vi "create_data_file.vi"   [LabVIEW 2019]
uses:
  Global Variables/global.vi
  Instrument_Setup.vi
  Global Variables/Data_Display_global.vi
  Global Variables/Heat_global_variables.vi
types:
  T1 = enum16{"open", "replace", "create", "open or create", "replace or create", "replace or create with confirmation"}
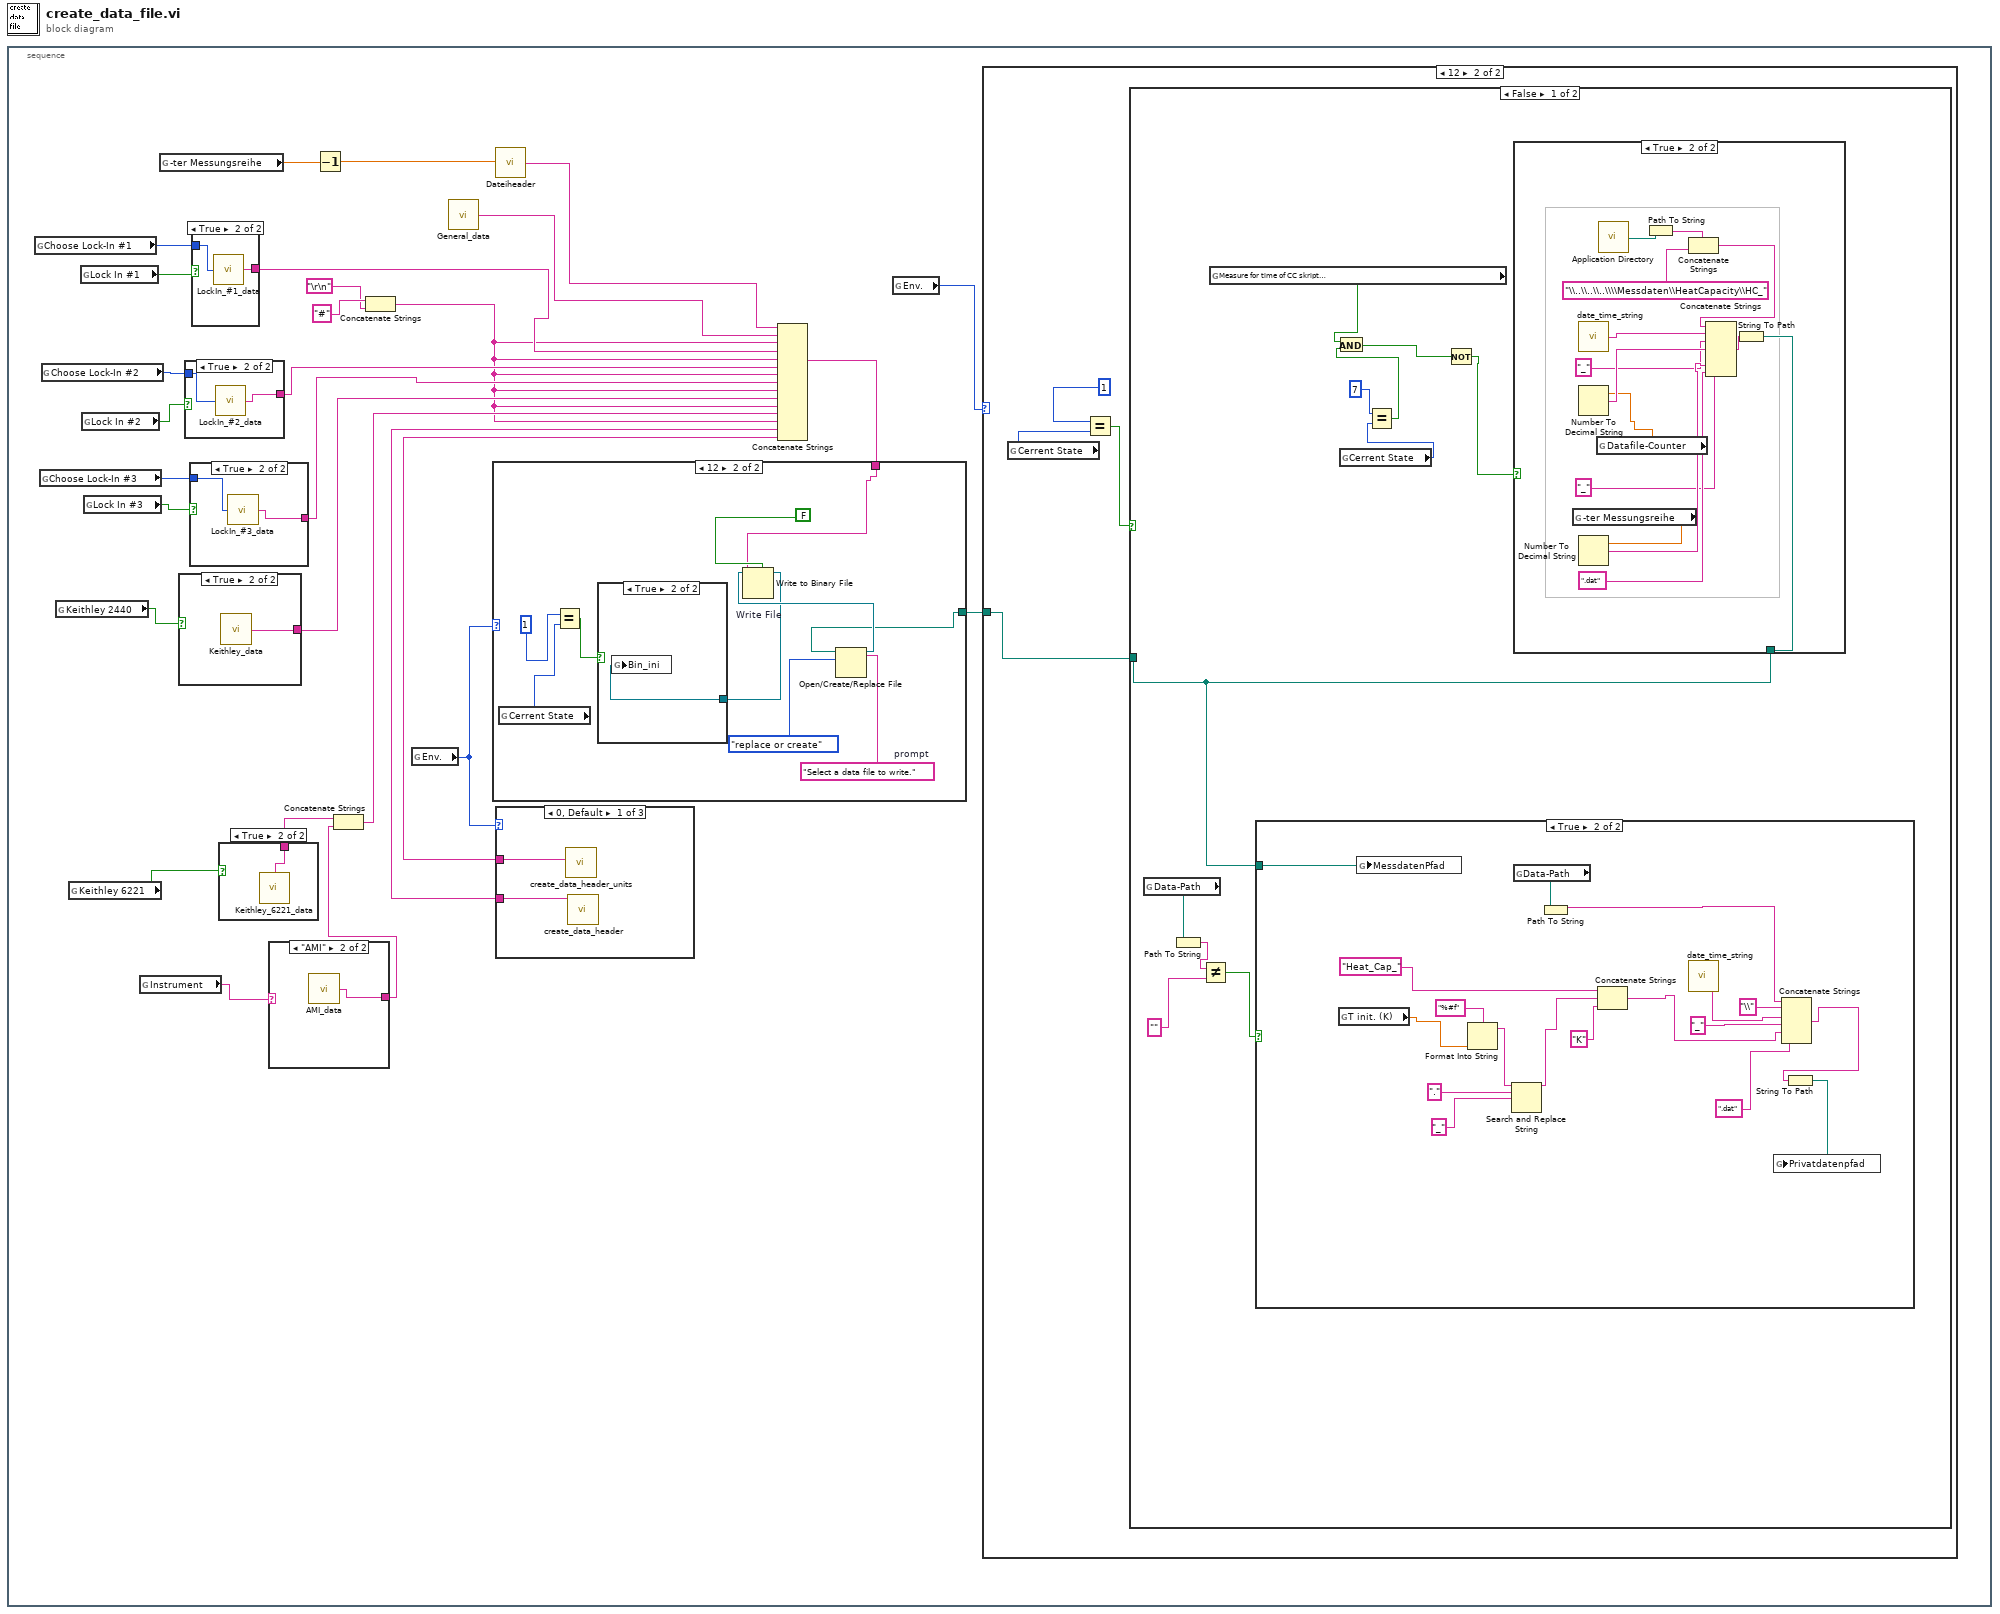
[diagram p0: block diagram]
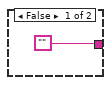
[diagram p2: hidden frame]
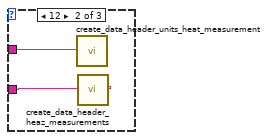
[diagram p3: hidden frame]
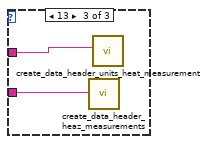
[diagram p4: hidden frame]
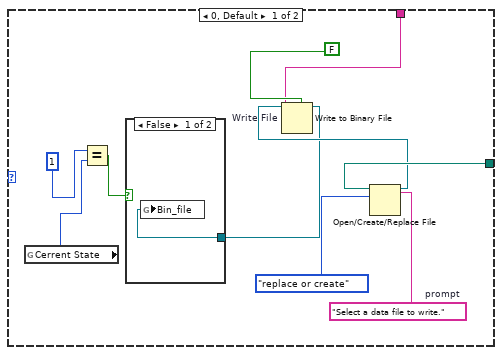
[diagram p5: hidden frame]
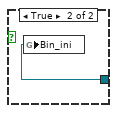
[diagram p6: hidden frame]
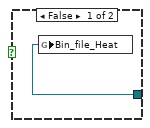
[diagram p7: hidden frame]
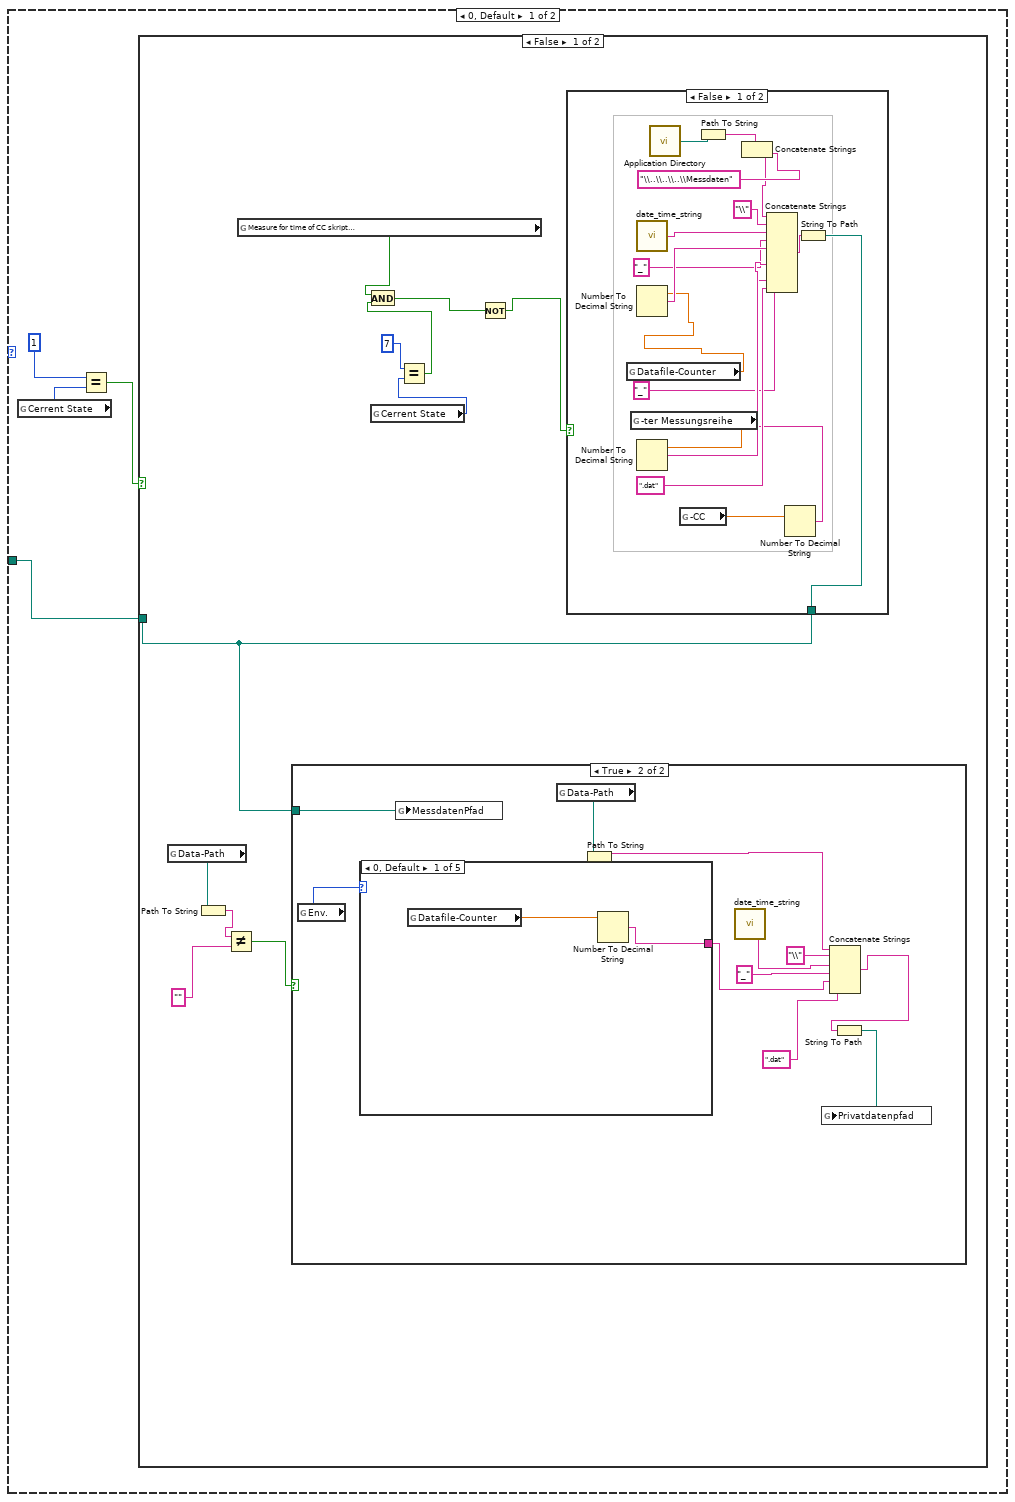
[diagram p8: hidden frame]
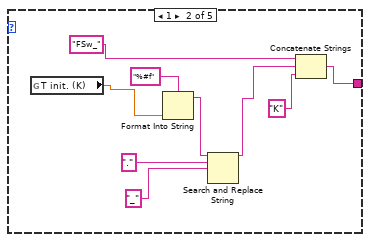
[diagram p10: hidden frame]
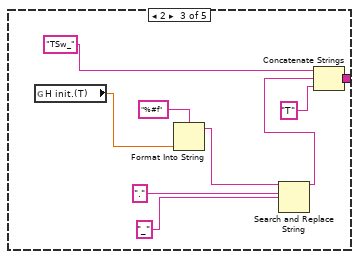
[diagram p11: hidden frame]
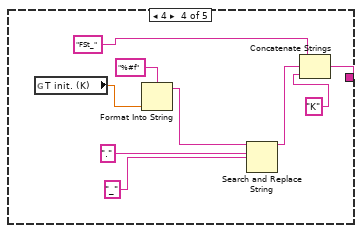
[diagram p12: hidden frame]
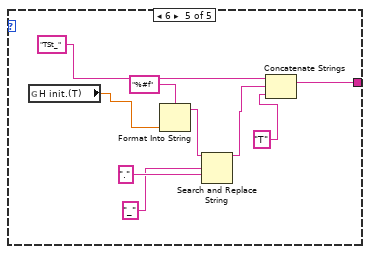
[diagram p13: hidden frame]
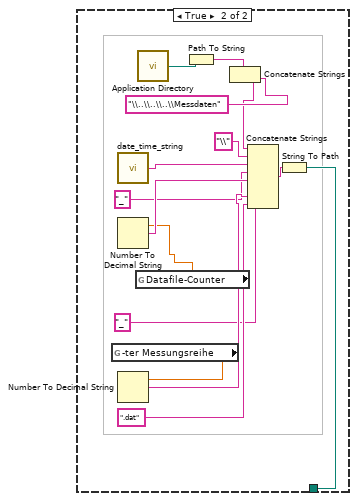
[diagram p14: hidden frame]
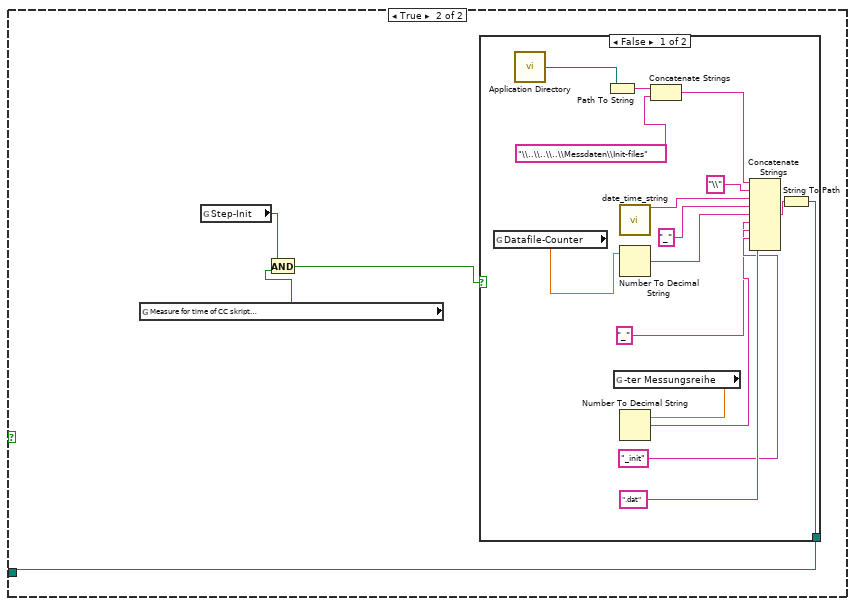
[diagram p15: hidden frame]
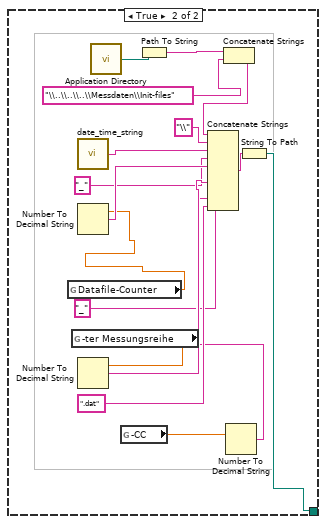
[diagram p16: hidden frame]
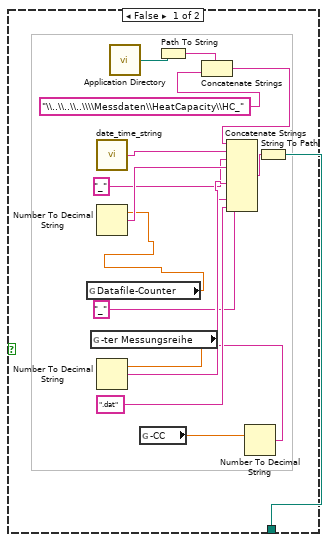
[diagram p18: hidden frame]
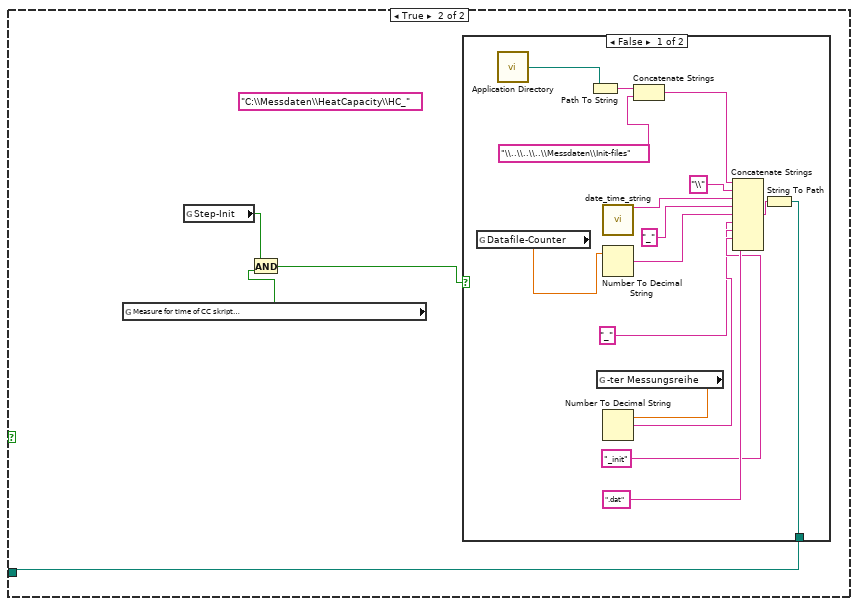
[diagram p19: hidden frame]
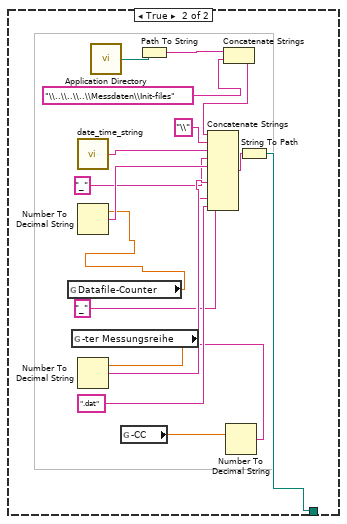
[diagram p20: hidden frame]
diagram:
  n1 = stacked-sequence {
    frame #0 {
      n2 = global read "Instrument_Setup.vi" "Choose Lock-In #1"() -> (w10:u16)
      n3 = global read "Instrument_Setup.vi" "Choose Lock-In #3"() -> (w7:u16)
      n4 = global read "Instrument_Setup.vi" "Choose Lock-In #2"() -> (w8:u16)
      n5 = global read "Instrument_Setup.vi" "Keithley 2440"() -> (w4:bool)
      n6 = global read "Instrument_Setup.vi" "Keithley 6221"() -> (w18:bool)
      n7 = global read "Instrument_Setup.vi" "Lock In #1"() -> (w21:bool)
      n8 = global read "Instrument_Setup.vi" "Lock In #2"() -> (w20:bool)
      n9 = global read "Instrument_Setup.vi" "Lock In #3"() -> (w12:bool)
      n10 = global read "Instrument_Setup.vi" "Instrument"() -> (w17:string)
      n11 = global read "global.vi" "-ter Messungsreihe"() -> (w26:dbl)
      n12 = case shown="True" w4 {
        tunnel: ["" w31] -> w13
        frame False {
        }
        frame True {
          n13 = call "Keithley_data.vi"() -> ("String"=w31:string)
        }
      }
      n14 = case shown="True" w20 {
        tunnel: ["" w304] -> w9
        tunnel: w8 -> [_ w303]
        frame False {
        }
        frame True {
          n15 = call "LockIn_#2_data.vi"("Choose Lock-In #3"=w303) -> ("String"=w304:string)
        }
      }
      n16 = case shown="True" w12 {
        tunnel: ["" w297] -> w11
        tunnel: w7 -> [_ w296]
        frame False {
        }
        frame True {
          n17 = call "LockIn_#3_data.vi"("Choose Lock-In #3"=w296) -> ("String"=w297:string)
        }
      }
      n18 = case shown="True" w21 {
        tunnel: ["" w307] -> w22
        tunnel: w10 -> [_ w306]
        frame False {
        }
        frame True {
          n19 = call "LockIn_#1_data.vi"("Choose Lock-In #3"=w306) -> ("String"=w307:string)
        }
      }
      n20 = case shown="True" w18 {
        tunnel: ["" w301] -> w16
        frame False {
        }
        frame True {
          n21 = call "Keithley_6221_data.vi"() -> ("String"=w301:string)
        }
      }
      n22 = case shown="\"AMI\"" w17 {
        tunnel: ["" w299] -> w15
        frame "Sweet 16", Default {
        }
        frame "AMI" {
          n23 = call "AMI_data.vi"() -> ("String"=w299:string)
        }
      }
      n24 = Decrement(x=w26) -> (x-1=w25:dbl)
      n25 = Concatenate Strings(w16, w15) -> (w14:string)
      n26 = Concatenate Strings("#", "\r\n") -> (w1:string)
      n27 = global read "global.vi" "Env."() -> (w5:i32)
      n28 = call "General_data.vi"() -> ("String"=w27:string)
      n29 = call "Dateiheader.vi"("Zeilenindex"=w25) -> ("String"=w28:string)
      n30 = case shown="0, Default" w5 {
        tunnel: [w33 w35 w36] -> w3
        tunnel: [w32 w34 w37] -> w2
        frame 0, Default {
          n31 = call "create_data_header_units.vi"() -> ("header units"=w33:string)  [unwired: 10 in]
          n32 = call "create_data_header.vi"() -> ("String"=w32:string)  [unwired: 11 in]
        }
        frame 12 {
          n33 = call "create_data_header_units_heat_measurement.vi"() -> ("header units"=w35:string)  [unwired: 11 in]
          n34 = call "create_data_header_heaz_measurements.vi"() -> ("data header"=w34:string)  [unwired: 11 in]
        }
        frame 13 {
          n35 = call "create_data_header_heaz_measurements.vi"() -> ("data header"=w37:string)  [unwired: 11 in]
          n36 = call "create_data_header_units_heat_measurement.vi"() -> ("header units"=w36:string)  [unwired: 11 in]
        }
      }
      n37 = Concatenate Strings(w28, w27, w1, w22, w1, w9, w1, w11, w1, w13, w1, w14, w1, w2, w3) -> (w19:string)
      n38 = global read "global.vi" "Env."() -> (w6:i32)
      n39 = case shown="12" w6 {
        tunnel: [w62 w195] -> w29
        frame 0, Default {
          n40 = global read "global.vi" "Cerrent State"() -> (w64:i32)
          n41 = Equal?(x=1, y=w64) -> (x = y?=w63:bool)
          n42 = case shown="False" w63 {
            tunnel: [w70 w161] -> w62
            frame False {
              n43 = global read "Instrument_Setup.vi" "Data-Path"() -> (w69:path)
              n44 = Path To String(path=w69) -> (string=w68:string)
              n45 = Not Equal?(x=w68, y="") -> (x != y?=w66:bool)
              n46 = global read "Instrument_Setup.vi" "Measure for time of CC skript\nat each field step point"() -> (w74:bool)
              n47 = global read "global.vi" "Cerrent State"() -> (w76:i32)
              n48 = Equal?(x=7, y=w76) -> (x = y?=w73:bool)
              n49 = And(x=w74, y=w73) -> (x .and. y?=w72:bool)
              n50 = Not(x=w72) -> (.not. x?=w71:bool)
              n51 = case shown="False" w71 {
                tunnel: [w135 w148] -> w70
                frame False {
                  w131 = "_"
                  n52 = global read "Data_Display_global.vi" "Datafile-Counter"() -> (w130:dbl)
                  n53 = global read "global.vi" "-ter Messungsreihe"() -> (w137:dbl)
                  n54 = call "date_time_string.vi"() -> ("date/time string"=w139:string)  [unwired: 1 in]
                  n55 = Number To Decimal String(number=w130) -> (decimal integer string=w141:string)  [unwired: 1 in]
                  n56 = Number To Decimal String(number=w137) -> (decimal integer string=w142:string)  [unwired: 1 in]
                  n57 = call <vilib>:"Application Directory.vi"() -> ("Application Directory"=w129:path)
                  n58 = global read "global.vi" "-CC"() -> (w133:dbl)
                  n59 = Path To String(path=w129) -> (string=w128:string)
                  n60 = Concatenate Strings(w128, "\\..\\..\\..\\Messdaten") -> (w126:string)
                  n61 = Number To Decimal String(number=w133) -> (decimal integer string=w132:string)  [unwired: 1 in]
                  n62 = Concatenate Strings(w126, "\\", w139, "_", w141, w131, w142, w131, w132, ".dat") -> (w136:string)
                  n63 = String To Path(string=w136) -> (path=w135:path)
                }
                frame True {
                  n64 = global read "global.vi" "-ter Messungsreihe"() -> (w150:dbl)
                  n65 = call "date_time_string.vi"() -> ("date/time string"=w152:string)  [unwired: 1 in]
                  n66 = Number To Decimal String(number=w150) -> (decimal integer string=w156:string)  [unwired: 1 in]
                  n67 = global read "Data_Display_global.vi" "Datafile-Counter"() -> (w147:dbl)
                  n68 = Number To Decimal String(number=w147) -> (decimal integer string=w154:string)  [unwired: 1 in]
                  n69 = call <vilib>:"Application Directory.vi"() -> ("Application Directory"=w146:path)
                  n70 = Path To String(path=w146) -> (string=w145:string)
                  n71 = Concatenate Strings(w145, "\\..\\..\\..\\Messdaten") -> (w143:string)
                  n72 = Concatenate Strings(w143, "\\", w152, "_", w154, "_", w156, ".dat") -> (w149:string)
                  n73 = String To Path(string=w149) -> (path=w148:path)
                }
              }
              n74 = case shown="True" w66 {
                tunnel: w70 -> [_ w80]
                frame False {
                }
                frame True {
                  n75 = global read "global.vi" "Env."() -> (w86:i32)
                  n76 = case shown="0, Default" w86 {
                    tunnel: [w88 w97 w106 w115 w124] -> w78
                    frame 0, Default {
                      n77 = global read "Data_Display_global.vi" "Datafile-Counter"() -> (w89:dbl)
                      n78 = Number To Decimal String(number=w89) -> (decimal integer string=w88:string)  [unwired: 1 in]
                    }
                    frame 1 {
                      n79 = global read "global.vi" "T init. (K)"() -> (w92:dbl)
                      n80 = Format Into String(format string="%#f", w92) -> (resulting string=w94:string)  [unwired: 2 in, 1 out]
                      n81 = Search and Replace String(input string=w94, search string=".", replace string="_") -> (result string=w93:string)  [unwired: 5 in, 3 out]
                      n82 = Concatenate Strings("FSw_", w93, "K") -> (w97:string)
                    }
                    frame 2 {
                      n83 = global read "global.vi" "H init.(T)"() -> (w101:dbl)
                      n84 = Format Into String(format string="%#f", w101) -> (resulting string=w103:string)  [unwired: 2 in, 1 out]
                      n85 = Search and Replace String(input string=w103, search string=".", replace string="_") -> (result string=w102:string)  [unwired: 5 in, 3 out]
                      n86 = Concatenate Strings("TSw_", w102, "T") -> (w106:string)
                    }
                    frame 4 {
                      n87 = global read "global.vi" "T init. (K)"() -> (w110:dbl)
                      n88 = Format Into String(format string="%#f", w110) -> (resulting string=w112:string)  [unwired: 2 in, 1 out]
                      n89 = Search and Replace String(input string=w112, search string=".", replace string="_") -> (result string=w111:string)  [unwired: 5 in, 3 out]
                      n90 = Concatenate Strings("FSt_", w111, "K") -> (w115:string)
                    }
                    frame 6 {
                      n91 = global read "global.vi" "H init.(T)"() -> (w120:dbl)
                      n92 = Format Into String(format string="%#f", w120) -> (resulting string=w121:string)  [unwired: 2 in, 1 out]
                      n93 = Search and Replace String(input string=w121, search string=".", replace string="_") -> (result string=w119:string)  [unwired: 5 in, 3 out]
                      n94 = Concatenate Strings("TSt_", w119, "T") -> (w124:string)
                    }
                  }
                  n95 = global write "Data_Display_global.vi" "MessdatenPfad"(w80) -> ()
                  n96 = global read "Instrument_Setup.vi" "Data-Path"() -> (w87:path)
                  n97 = Path To String(path=w87) -> (string=w83:string)
                  n98 = call "date_time_string.vi"() -> ("date/time string"=w84:string)  [unwired: 1 in]
                  n99 = Concatenate Strings(w83, "\\", w84, "_", w78, ".dat") -> (w82:string)
                  n100 = String To Path(string=w82) -> (path=w81:path)
                  n101 = global write "Data_Display_global.vi" "Privatdatenpfad"(w81) -> ()
                }
              }
            }
            frame True {
              n102 = global read "Instrument_Setup.vi" "Measure for time of CC skript\nat each field step point"() -> (w159:bool)
              n103 = global read "global.vi" "Step-Init"() -> (w160:bool)
              n104 = And(x=w160, y=w159) -> (x .and. y?=w158:bool)
              n105 = case shown="False" w158 {
                tunnel: [w167 w178] -> w161
                frame False {
                  n106 = global read "Data_Display_global.vi" "Datafile-Counter"() -> (w166:dbl)
                  n107 = call <vilib>:"Application Directory.vi"() -> ("Application Directory"=w165:path)
                  n108 = Path To String(path=w165) -> (string=w164:string)
                  n109 = global read "global.vi" "-ter Messungsreihe"() -> (w169:dbl)
                  n110 = call "date_time_string.vi"() -> ("date/time string"=w171:string)  [unwired: 1 in]
                  n111 = Number To Decimal String(number=w166) -> (decimal integer string=w173:string)  [unwired: 1 in]
                  n112 = Number To Decimal String(number=w169) -> (decimal integer string=w175:string)  [unwired: 1 in]
                  n113 = Concatenate Strings(w164, "\\..\\..\\..\\Messdaten\\Init-files") -> (w162:string)
                  n114 = Concatenate Strings(w162, "\\", w171, "_", w173, "_", w175, "_init", ".dat") -> (w168:string)
                  n115 = String To Path(string=w168) -> (path=w167:path)
                }
                frame True {
                  w184 = "_"
                  n116 = global read "Data_Display_global.vi" "Datafile-Counter"() -> (w183:dbl)
                  n117 = global read "global.vi" "-ter Messungsreihe"() -> (w189:dbl)
                  n118 = call "date_time_string.vi"() -> ("date/time string"=w191:string)  [unwired: 1 in]
                  n119 = Number To Decimal String(number=w183) -> (decimal integer string=w193:string)  [unwired: 1 in]
                  n120 = Number To Decimal String(number=w189) -> (decimal integer string=w194:string)  [unwired: 1 in]
                  n121 = call <vilib>:"Application Directory.vi"() -> ("Application Directory"=w182:path)
                  n122 = global read "global.vi" "-CC"() -> (w186:dbl)
                  n123 = Path To String(path=w182) -> (string=w181:string)
                  n124 = Concatenate Strings(w181, "\\..\\..\\..\\Messdaten\\Init-files") -> (w179:string)
                  n125 = Number To Decimal String(number=w186) -> (decimal integer string=w185:string)  [unwired: 1 in]
                  n126 = Concatenate Strings(w179, "\\", w191, "_", w193, w184, w194, w184, w185, ".dat") -> (w188:string)
                  n127 = String To Path(string=w188) -> (path=w178:path)
                }
              }
            }
          }
        }
        frame 12 {
          n128 = global read "global.vi" "Cerrent State"() -> (w197:i32)
          n129 = Equal?(x=1, y=w197) -> (x = y?=w196:bool)
          n130 = case shown="False" w196 {
            tunnel: [w203 w261] -> w195
            frame False {
              n131 = global read "Instrument_Setup.vi" "Data-Path"() -> (w202:path)
              n132 = Path To String(path=w202) -> (string=w201:string)
              n133 = Not Equal?(x=w201, y="") -> (x != y?=w199:bool)
              n134 = global read "Instrument_Setup.vi" "Measure for time of CC skript\nat each field step point"() -> (w207:bool)
              n135 = global read "global.vi" "Cerrent State"() -> (w209:i32)
              n136 = Equal?(x=7, y=w209) -> (x = y?=w206:bool)
              n137 = And(x=w207, y=w206) -> (x .and. y?=w205:bool)
              n138 = Not(x=w205) -> (.not. x?=w204:bool)
              n139 = case shown="True" w204 {
                tunnel: [w237 w249] -> w203
                frame False {
                  w233 = "_"
                  n140 = global read "Data_Display_global.vi" "Datafile-Counter"() -> (w232:dbl)
                  n141 = global read "global.vi" "-ter Messungsreihe"() -> (w239:dbl)
                  n142 = call "date_time_string.vi"() -> ("date/time string"=w240:string)  [unwired: 1 in]
                  n143 = Number To Decimal String(number=w232) -> (decimal integer string=w242:string)  [unwired: 1 in]
                  n144 = Number To Decimal String(number=w239) -> (decimal integer string=w243:string)  [unwired: 1 in]
                  n145 = call <vilib>:"Application Directory.vi"() -> ("Application Directory"=w231:path)
                  n146 = global read "global.vi" "-CC"() -> (w235:dbl)
                  n147 = Path To String(path=w231) -> (string=w230:string)
                  n148 = Concatenate Strings(w230, "\\..\\..\\..\\\\Messdaten\\HeatCapacity\\HC_") -> (w228:string)
                  n149 = Number To Decimal String(number=w235) -> (decimal integer string=w234:string)  [unwired: 1 in]
                  n150 = Concatenate Strings(w228, w240, "_", w242, w233, w243, w233, w234, ".dat") -> (w238:string)
                  n151 = String To Path(string=w238) -> (path=w237:path)
                }
                frame True {
                  n152 = global read "global.vi" "-ter Messungsreihe"() -> (w251:dbl)
                  n153 = call "date_time_string.vi"() -> ("date/time string"=w252:string)  [unwired: 1 in]
                  n154 = Number To Decimal String(number=w251) -> (decimal integer string=w256:string)  [unwired: 1 in]
                  n155 = global read "Data_Display_global.vi" "Datafile-Counter"() -> (w248:dbl)
                  n156 = Number To Decimal String(number=w248) -> (decimal integer string=w254:string)  [unwired: 1 in]
                  n157 = call <vilib>:"Application Directory.vi"() -> ("Application Directory"=w247:path)
                  n158 = Path To String(path=w247) -> (string=w246:string)
                  n159 = Concatenate Strings(w246, "\\..\\..\\..\\\\Messdaten\\HeatCapacity\\HC_") -> (w244:string)
                  n160 = Concatenate Strings(w244, w252, "_", w254, "_", w256, ".dat") -> (w250:string)
                  n161 = String To Path(string=w250) -> (path=w249:path)
                }
              }
              n162 = case shown="True" w199 {
                tunnel: w203 -> [_ w221]
                frame False {
                }
                frame True {
                  n163 = global read "global.vi" "T init. (K)"() -> (w213:dbl)
                  n164 = global write "Data_Display_global.vi" "MessdatenPfad"(w221) -> ()
                  n165 = Format Into String(format string="%#f", w213) -> (resulting string=w215:string)  [unwired: 2 in, 1 out]
                  n166 = Search and Replace String(input string=w215, search string=".", replace string="_") -> (result string=w214:string)  [unwired: 5 in, 3 out]
                  n167 = global read "Instrument_Setup.vi" "Data-Path"() -> (w227:path)
                  n168 = Path To String(path=w227) -> (string=w224:string)
                  n169 = Concatenate Strings("Heat_Cap_", w214, "K") -> (w210:string)
                  n170 = call "date_time_string.vi"() -> ("date/time string"=w225:string)  [unwired: 1 in]
                  n171 = Concatenate Strings(w224, "\\", w225, "_", w210, ".dat") -> (w223:string)
                  n172 = String To Path(string=w223) -> (path=w222:path)
                  n173 = global write "Data_Display_global.vi" "Privatdatenpfad"(w222) -> ()
                }
              }
            }
            frame True {
              (unwired) "C:\\Messdaten\\HeatCapacity\\HC_"
              n174 = global read "Instrument_Setup.vi" "Measure for time of CC skript\nat each field step point"() -> (w259:bool)
              n175 = global read "global.vi" "Step-Init"() -> (w260:bool)
              n176 = And(x=w260, y=w259) -> (x .and. y?=w258:bool)
              n177 = case shown="False" w258 {
                tunnel: [w267 w278] -> w261
                frame False {
                  n178 = global read "Data_Display_global.vi" "Datafile-Counter"() -> (w266:dbl)
                  n179 = call <vilib>:"Application Directory.vi"() -> ("Application Directory"=w265:path)
                  n180 = Path To String(path=w265) -> (string=w264:string)
                  n181 = global read "global.vi" "-ter Messungsreihe"() -> (w269:dbl)
                  n182 = call "date_time_string.vi"() -> ("date/time string"=w271:string)  [unwired: 1 in]
                  n183 = Number To Decimal String(number=w266) -> (decimal integer string=w273:string)  [unwired: 1 in]
                  n184 = Number To Decimal String(number=w269) -> (decimal integer string=w275:string)  [unwired: 1 in]
                  n185 = Concatenate Strings(w264, "\\..\\..\\..\\Messdaten\\Init-files") -> (w262:string)
                  n186 = Concatenate Strings(w262, "\\", w271, "_", w273, "_", w275, "_init", ".dat") -> (w268:string)
                  n187 = String To Path(string=w268) -> (path=w267:path)
                }
                frame True {
                  w284 = "_"
                  n188 = global read "Data_Display_global.vi" "Datafile-Counter"() -> (w283:dbl)
                  n189 = global read "global.vi" "-ter Messungsreihe"() -> (w289:dbl)
                  n190 = call "date_time_string.vi"() -> ("date/time string"=w291:string)  [unwired: 1 in]
                  n191 = Number To Decimal String(number=w283) -> (decimal integer string=w293:string)  [unwired: 1 in]
                  n192 = Number To Decimal String(number=w289) -> (decimal integer string=w294:string)  [unwired: 1 in]
                  n193 = call <vilib>:"Application Directory.vi"() -> ("Application Directory"=w282:path)
                  n194 = global read "global.vi" "-CC"() -> (w286:dbl)
                  n195 = Path To String(path=w282) -> (string=w281:string)
                  n196 = Concatenate Strings(w281, "\\..\\..\\..\\Messdaten\\Init-files") -> (w279:string)
                  n197 = Number To Decimal String(number=w286) -> (decimal integer string=w285:string)  [unwired: 1 in]
                  n198 = Concatenate Strings(w279, "\\", w291, "_", w293, w284, w294, w284, w285, ".dat") -> (w288:string)
                  n199 = String To Path(string=w288) -> (path=w278:path)
                }
              }
            }
          }
        }
      }
      n200 = case shown="12" w5 {
        tunnel: w29 -> [w46 w50]
        tunnel: w19 -> [w39 w51]
        frame 0, Default {
          w47 = "Select a data file to write."  # prompt
          n201 = global read "global.vi" "Cerrent State"() -> (w44:i32)
          n202 = Equal?(x=1, y=w44) -> (x = y?=w43:bool)
          n203 = Open/Create/Replace File(file path (use dialog)=w46, prompt=w47, operation (0:open)=T1."replace or create") -> (refnum out=w42:refnum<file>)  [unwired: 3 in, 2 out]
          n204 = Write to Binary File "Write File"(file (use dialog)=w42, data=w39, 5:FALSE ("prepend array or string size? (T)")) -> (refnum out=w41:refnum<file>)  [unwired: 3 in, 2 out]
          n205 = case shown="False" w43 {
            tunnel: w41 -> [w48 w49]
            frame False {
              n206 = global write "Instrument_Setup.vi" "Bin_file"(w48) -> ()
            }
            frame True {
              n207 = global write "Instrument_Setup.vi" "Bin_ini"(w49) -> ()
            }
          }
        }
        frame 12 {
          w59 = "Select a data file to write."  # prompt
          n208 = global read "global.vi" "Cerrent State"() -> (w57:i32)
          n209 = Equal?(x=1, y=w57) -> (x = y?=w56:bool)
          n210 = Open/Create/Replace File(file path (use dialog)=w50, prompt=w59, operation (0:open)=T1."replace or create") -> (refnum out=w55:refnum<file>)  [unwired: 3 in, 2 out]
          n211 = Write to Binary File "Write File"(file (use dialog)=w55, data=w51, 5:FALSE ("prepend array or string size? (T)")) -> (refnum out=w54:refnum<file>)  [unwired: 3 in, 2 out]
          n212 = case shown="True" w56 {
            tunnel: w54 -> [w60 w61]
            frame False {
              n213 = global write "Heat_global_variables.vi" "Bin_file_Heat"(w60) -> ()
            }
            frame True {
              n214 = global write "Instrument_Setup.vi" "Bin_ini"(w61) -> ()
            }
          }
        }
      }
    }
  }
